vi "Get Object Status.vi"(8 "error in (no error)":errorcluster, 11 "Instrument in":refnum<class "Instrument.lvclass">) -> (0 "error out":errorcluster, 2 "Status":bool, 3 "Instrument out":refnum<class "Instrument.lvclass">)   [LabVIEW 2015]
uses:
  Instrument.lvclass
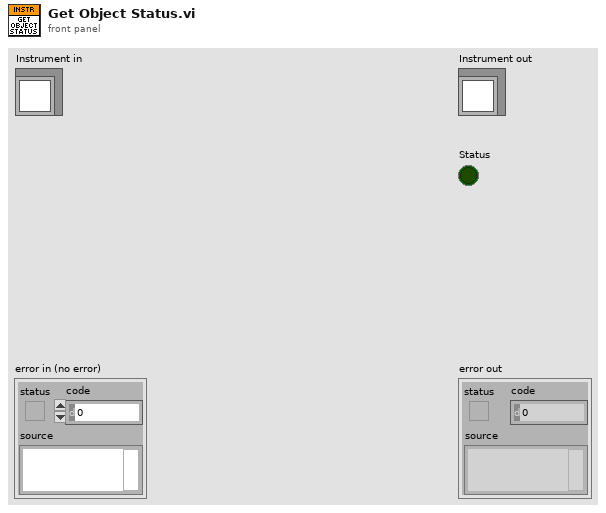
[diagram p1: front panel]
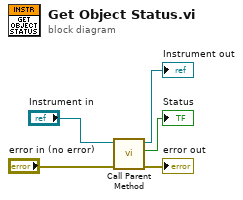
[diagram p0: block diagram]
diagram:
  n1 = call-parent "Call Parent Method"("error in (no error)"="error in (no error)", "Base Class in"="Instrument in") -> ("error out"=→"error out":errorcluster, "Status"=→"Status":bool, "Base Class out"=→"Instrument out":refnum<class "Instrument.lvclass">)  [unwired: 7 in]
